vi "SPI Write Read Bits.vi"(6 "ReadBitsNum":i32, 7 "pReadBitStr":string, 9 "pWriteBitStr":string, 10 "SPIIndex":i32, 11 "DevHandle":i32) -> (1 "pWriteBitStr out":string, 3 "function return":i32, 5 "pReadBitStr out":string)   [LabVIEW 2010, in "usb2spi.lvlib"]
doc: "int WINAPI SPI_WriteReadBits(int DevHandle,int SPIIndex,char *pWriteBitStr,char *pReadBitStr,int ReadBitsNum);"
uses:
  usb2spi.lvlib
  USB2XXX.dll
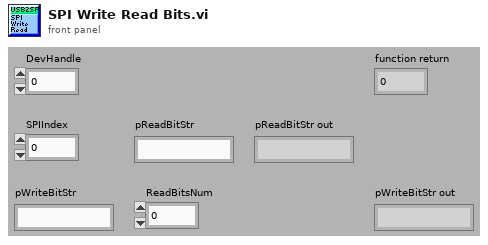
[diagram p1: front panel]
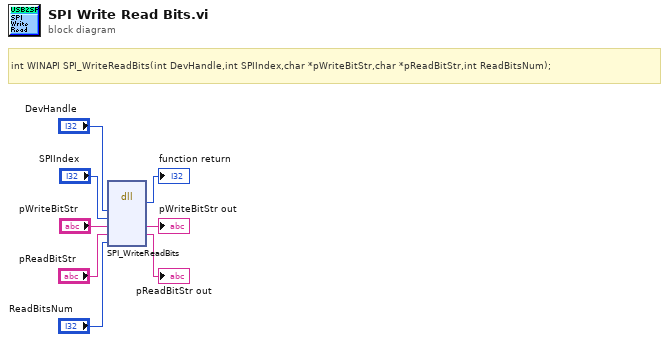
[diagram p0: block diagram]
diagram:
  # "int WINAPI SPI_WriteReadBits(int DevHandle,int SPIIndex,char *pWriteBitStr,char *pReadBitStr,int ReadBitsNum);"
  n1 = dll-call lib="G:/OtherWork/USB2XXX_Example/trunk/Labview/PublicFiles/usb2spi/USB2XXX.*" fn="SPI_WriteReadBits"("DevHandle"="DevHandle", "SPIIndex"="SPIIndex", "pWriteBitStr"="pWriteBitStr", "pReadBitStr"="pReadBitStr", "ReadBitsNum"="ReadBitsNum") -> (→"function return":i32, "pWriteBitStr"=→"pWriteBitStr out":string, "pReadBitStr"=→"pReadBitStr out":string)  [unwired: 6 in, 2 out]
